vi "Unflatten Value.vi"(8 "error in (no error)":errorcluster, 10 "Value":string, 11 "Data Type in":refnum<class "Data Type.lvclass">) -> (0 "error out":errorcluster, 3 "Data Type out":refnum<class "Data Type.lvclass">)   [LabVIEW 2020, in "Data Type.lvclass"]
uses:
  <vilib>/gpm_packages/@cs/data-type-serializer/source/Data Type/Data Type.lvclass
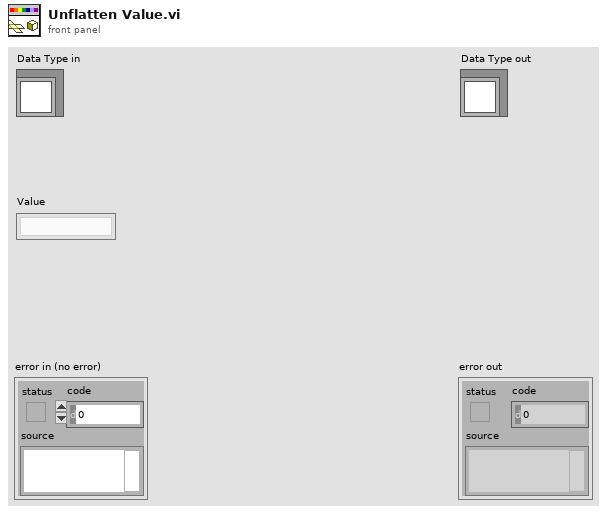
[diagram p1: front panel]
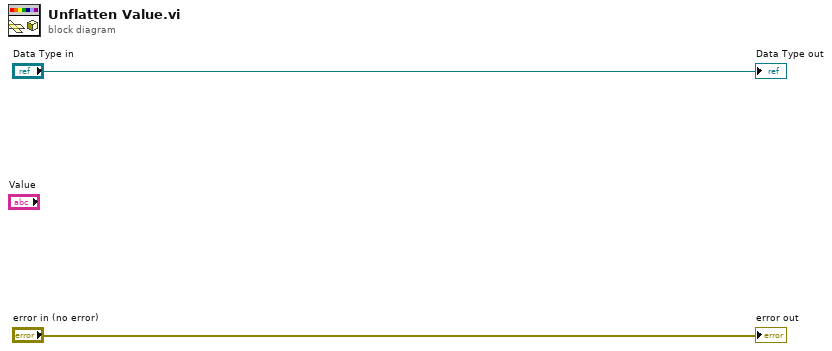
[diagram p0: block diagram]
diagram:
  "error out" <- "error in (no error)"
  "Data Type out" <- "Data Type in"
